vi "Execute Loaded Commands.vi"(8 "error in (no error)":errorcluster, 10 "Commands to Execute":i32=-1, 11 "Command Handler in":refnum<class "Command Handler.lvclass">) -> (0 "error out":errorcluster, 3 "Command Handler out":refnum<class "Command Handler.lvclass">)   [LabVIEW 2017, in "Command Handler.lvlib" / "Command Handler.lvclass"]
uses:
  Command Handler.lvclass
  Command Handler Messages/Command Handler Global API/Command Handler Global.vi
  Command Handler.lvlib
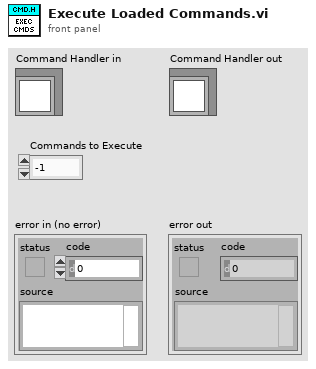
[diagram p1: front panel]
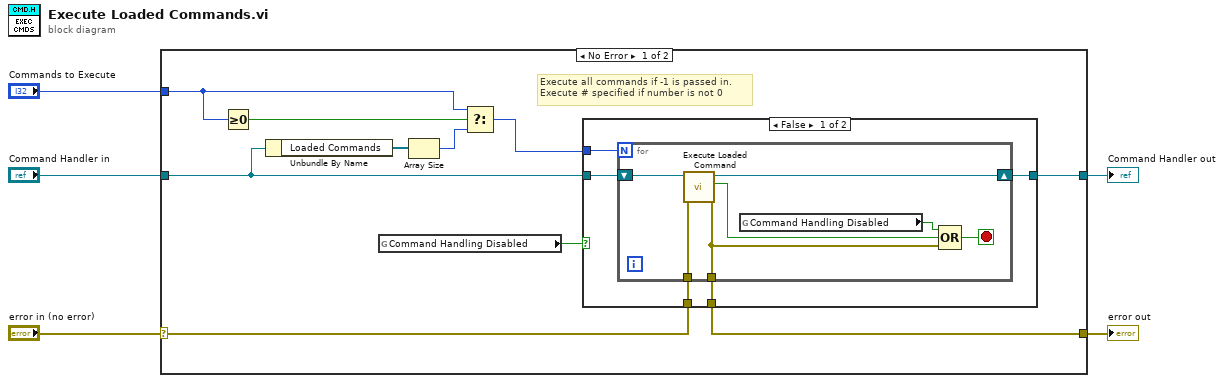
[diagram p0: block diagram]
diagram:
  n1 = case shown="No Error" "error in (no error)" {
    selector: "error in (no error)" -> [w15 w31]
    tunnel: [w14 w31] -> w4
    tunnel: [w13 w30] -> w2
    tunnel: "Command Handler in" -> [w12 w30]
    tunnel: "Commands to Execute" -> [w9 _]
    frame No Error {
      # "Execute all commands if -1 is passed in. \nExecute # specified if number is not 0"
      n2 = Greater Or Equal To 0?(x=w9) -> (x >= 0?=w10:bool)
      n3 = Unbundle By Name(w12) -> ("Loaded Commands"=w11:refnum<class "Command.lvclass">[])
      n4 = global read "Command Handler Global.vi" "Command Handling Disabled"() -> (w6:bool)
      n5 = Array Size(array=w11) -> (size(s)=w8:i32)
      n6 = Select(t=w9, s=w10, f=w8) -> (s? t:f=w7:i32)
      n7 = case shown="False" w6 {
        tunnel: w15 -> [w20 w29]
        tunnel: [w19 w29] -> w14
        tunnel: [w18 w28] -> w13
        tunnel: w12 -> [w17 w28]
        tunnel: w7 -> [w16 _]
        frame False {
          n8 = for {
            N: w16 -> [_]
            tunnel: w20 -> [w25]
            tunnel: [w23] -> w19
            shift-right: [w26] -> w18
            shift-left: w17 -> [w27]
            stop <- w22 stop-if-true
            n9 = call-dynamic "Execute Loaded Command.vi"("error in (no error)"=w25, "Command Handler in"=w27) -> ("error out"=w23:errorcluster, "Stop"=w24:bool, "Command Handler out"=w26:refnum<class "Command Handler.lvclass">)  [unwired: 7 in]
            n10 = global read "Command Handler Global.vi" "Command Handling Disabled"() -> (w21:bool)
            n11 = Compound Arithmetic op=OR(w21, w24, w23) -> (w22:bool)
          }
        }
        frame True {
        }
      }
    }
    frame Error {
    }
  }
  "error out" <- w4
  "Command Handler out" <- w2
